vi "MBwaitForSerialDigStatus.vi"(10 "No. of points(1)":i32=1, 11 "Serial port (0)":i32) -> (1 "CRC":u16, 2 "Digital status":bool[](array[boolean]), 3 "String read":string)   [LabVIEW 2010]
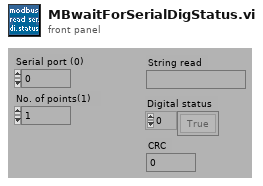
[diagram p1: front panel]
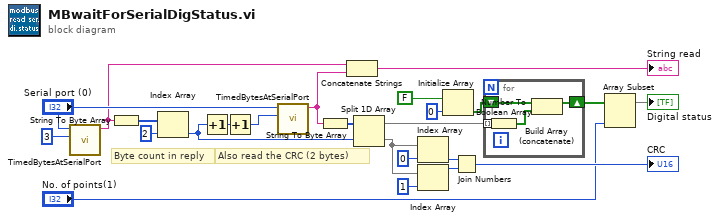
[diagram p0: block diagram]
diagram:
  # "Also read the CRC (2 bytes)"
  # "Byte count in reply"
  n1 = call "TimedBytesAtSerialPort.vi"("Byte count"=u32 3, "Serial port (0)"="Serial port (0)") -> ("String read"=w18:string)  [unwired: 1 in, 8 out]
  n2 = String To Byte Array(string=w18) -> (unsigned byte array=w22:u8[])
  n3 = Index Array(array=w22, index=2) -> (element=w15:u8)
  n4 = Increment(x=w15) -> (x+1=w21:u8)
  n5 = Increment(x=w21) -> (x+1=w20:u8)
  n6 = call "TimedBytesAtSerialPort.vi"("Byte count"=w20, "Serial port (0)"="Serial port (0)") -> ("String read"=w14:string)  [unwired: 1 in, 8 out]
  n7 = String To Byte Array(string=w14) -> (unsigned byte array=w16:u8[])
  n8 = Concatenate Strings(w18, w14) -> (→"String read":string)
  n9 = Split 1D Array(array=w16, index=w15) -> (first subarray=w4:u8[], second subarray=w9:u8[])
  n10 = Index Array(array=w9, index=0) -> (element=w12:u8)
  n11 = Index Array(array=w9, index=1) -> (element=w13:u8)
  n12 = Initialize Array(FALSE, 0) -> (w5:bool[])
  n13 = Join Numbers(hi=w12, lo=w13) -> ((hi.lo)=→"CRC":u16)
  n14 = for {
    shift-right: [w25] -> w2
    shift-left: w5 -> [w26]
    tunnel: w4 -> [w28] mode=indexing
    n15 = Number To Boolean Array(number=w28) -> (Boolean array=w27:bool[])
    n16 = Build Array (concatenate)(w26, w27) -> (w25:bool[])
  }
  n17 = Array Subset(array=w2, length="No. of points(1)") -> (→"Digital status":bool[])  [unwired: 1 in]
